vi "mqttTCPIPdisconnect.vi"(0 "mqtt in":refnum<class "mqtt.lvclass">, 11 "error in (no error)":errorcluster) -> (4 "mqtt out":refnum<class "mqtt.lvclass">, 15 "error out":errorcluster)   [LabVIEW 2017, in "mqtt.lvclass"]
uses:
  mqtt.lvclass
  mqtt.lvclass/mqtt.ctl
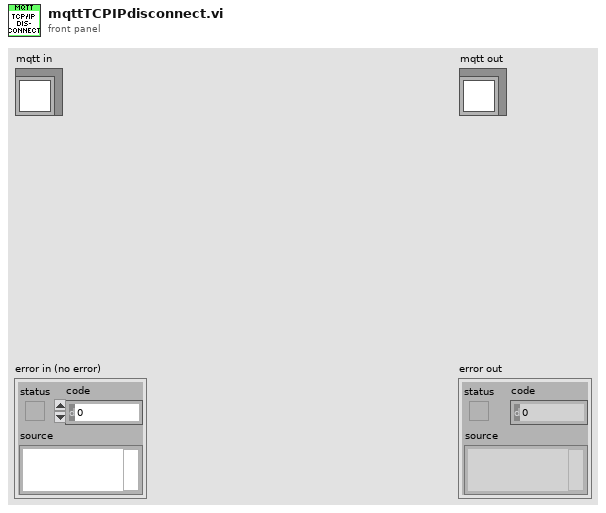
[diagram p1: front panel]
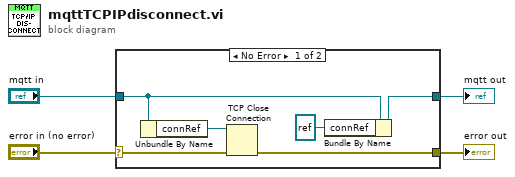
[diagram p0: block diagram]
diagram:
  n1 = case shown="No Error" "error in (no error)" {
    selector: "error in (no error)" -> [w10 w12]
    tunnel: [w9 w12] -> w3
    tunnel: [w5 w11] -> w1
    tunnel: "mqtt in" -> [w7 w11]
    frame No Error {
      n2 = Unbundle By Name(w7) -> ("connRef"=w8:refnum<k5>)
      n3 = TCP Close Connection(connection ID=w8, error in (no error)=w10) -> (error out=w9:errorcluster)  [unwired: 1 in, 1 out]
      n4 = Bundle By Name(cluster=w7, "connRef"=refnum<k5> refnum) -> (w5:refnum<class "mqtt.lvclass">)
    }
    frame Error {
    }
  }
  "error out" <- w3
  "mqtt out" <- w1
